vi "From CSV File.vi"(8 "error in":errorcluster, 9 "Path":path, 10 "engine in":refnum<class "engine configuration.lvclass">, 11 "SystemLink editor node in":refnum<class "SystemLink File editor node.lvclass">) -> (0 "error out":errorcluster, 1 "Update":bool, 2 "engine out":refnum<class "engine configuration.lvclass">, 3 "SystemLink editor node out":refnum<class "SystemLink File editor node.lvclass">)   [LabVIEW 2015, in "SystemLink File editor node.lvclass"]
uses:
  SystemLink File editor node.lvclass
  <vilib>/NI/Configuration Framework/serializable configuration/NISE_CEF_serializable configuration.lvclass
  <vilib>/NI/Module Execution Interface/Engine Configuration/engine configuration.lvclass
  <vilib>/NI/Tag Bus/tag/tag descriptor.lvclass
  module/configuration/SystemLink File configuration.lvclass
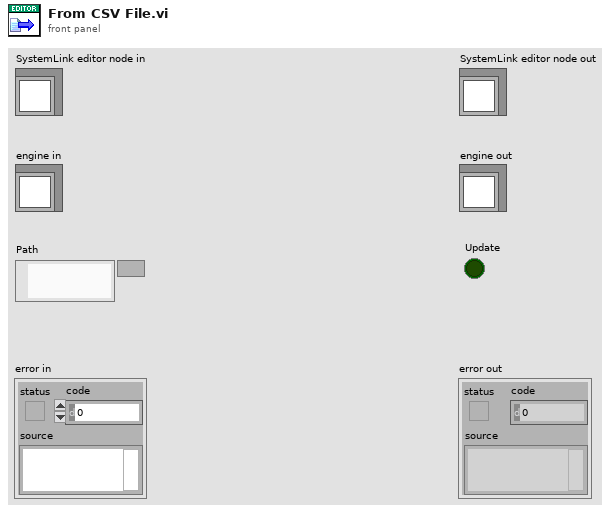
[diagram p1: front panel]
types:
  T1 = typedef "SystemLink File configuration.lvclass/Line.ctl" = cluster{"channel":refnum<class "TBM channel.lvclass">, "Data Tag Type":T2}
  T2 = typedef "SystemLink File configuration.lvclass/Data Tag Type.ctl" = enum16{"Double", "Single", "I32", "I16", "I8", "U64", "U32", "U16", "U8", "Boolean", "String", "Timestamp"}
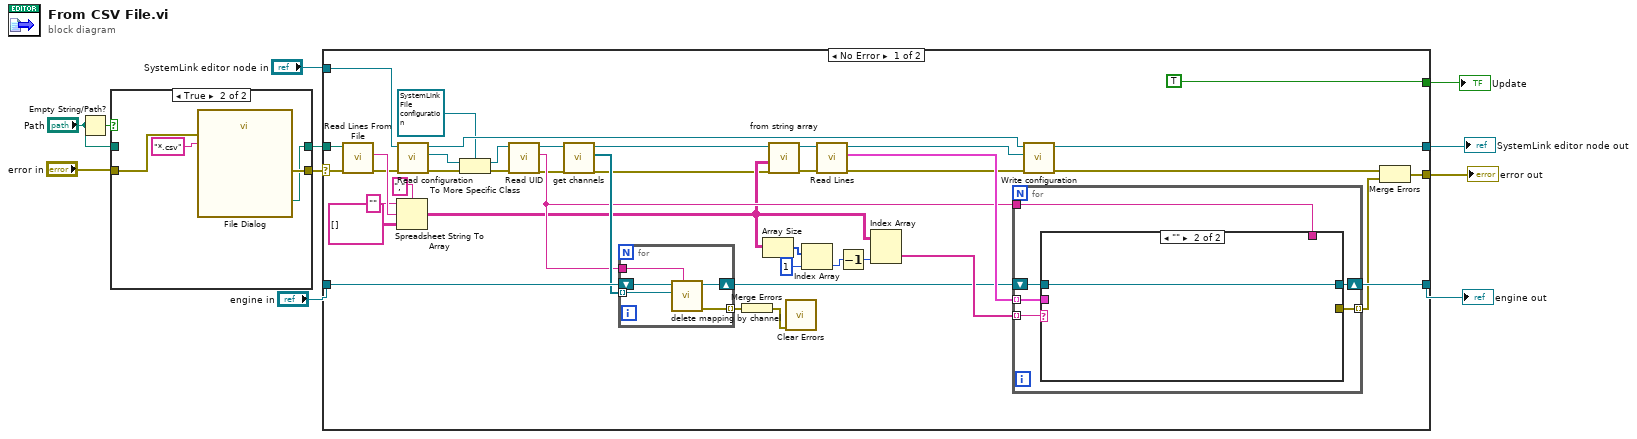
[diagram p0: block diagram]
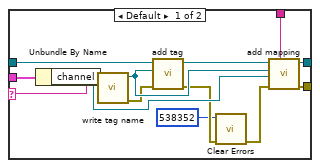
[diagram p3: hidden frame]
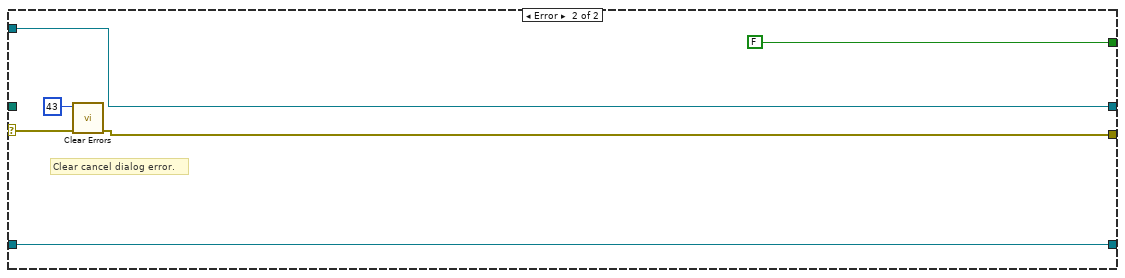
[diagram p4: hidden frame]
diagram:
  n1 = Empty String/Path?(string/path="Path") -> (empty?=w5:bool)
  n2 = case shown="True" w5 {
    tunnel: "error in" -> [w12 w16]
    tunnel: [w12 w15] -> w3
    tunnel: [w13 w14] -> w2
    tunnel: "Path" -> [w13 _]
    frame False {
    }
    frame True {
      n3 = call "File Dialog"("error in"=w16, "pattern (all files)"="*.csv") -> ("selected path"=w14:path, "error out"=w15:errorcluster)  [unwired: 10 in, 2 out]
    }
  }
  n4 = case shown="No Error" w3 {
    selector: w3 -> [w51 w86]
    tunnel: [w36 w85] -> w8
    tunnel: [w22 w88] -> w10
    tunnel: "SystemLink editor node in" -> [w29 w88]
    tunnel: w2 -> [w56 _]
    tunnel: [TRUE ("Update") FALSE ("Update")] -> w11
    tunnel: "engine in" -> [w48 w83]
    tunnel: [w39 w83] -> w9
    frame No Error {
      n5 = call <vilib>:"Read Lines From File.vi"("file path (dialog if empty)"=w56, "error in (not an error)"=w51) -> ("line string"=w54:string, "error out"=w28:errorcluster)  [unwired: 5 in, 1 out]
      n6 = Spreadsheet String To Array(delimiter (Tab)=",", format string="", spreadsheet string=w54, array type (2D Dbl)=string[][] [] ("type (empty)")) -> (array=w34:string[][])
      n7 = call-dynamic "Read configuration.vi"("error in"=w28, "SystemLin Tag Module editor node in"=w29) -> ("error out"=w26:errorcluster, "configuration"=w27:refnum<class "NISE_CEF_serializable configuration.lvclass">, "SystemLin Tag Module editor node out"=w25:refnum<class "SystemLink File editor node.lvclass">)  [unwired: 7 in]
      n8 = To More Specific Class(target class=refnum<class "SystemLink File configuration.lvclass"> refnum ("SystemLin Tag Module configuration"), reference=w27, error in=w26) -> (specific class reference=w50:refnum<class "SystemLink File configuration.lvclass">, error out=w44:errorcluster)
      n9 = call <vilib>:"Read UID.vi"("error in"=w44, "configuration in"=w50) -> ("error out"=w19:errorcluster, "instance id"=w37:string, "configuration out"=w49:refnum<class "SystemLink File configuration.lvclass">)  [unwired: 7 in]
      n10 = call-dynamic "get channels.vi"("SystemLin Tag Module configuration in"=w49) -> ("channels"=w47:refnum<class "TBM channel.lvclass">[], "SystemLin Tag Module configuration out"=w45:refnum<class "SystemLink File configuration.lvclass">)  [unwired: 9 in]
      n11 = for {
        tunnel: w37 -> [w81]
        tunnel: w47 -> [w80] mode=indexing
        tunnel: [w79] -> w46 mode=indexing
        shift-right: [w78] -> w40
        shift-left: w48 -> [w82]
        n12 = call <vilib>:"delete mapping by channel.vi"("owner ID"=w81, "channel"=w80, "engine configuration in"=w82) -> ("error out"=w79:errorcluster, "engine configuration out"=w78:refnum<class "engine configuration.lvclass">)  [unwired: 7 in]
      }
      n13 = Merge Errors(w46) -> (w20:errorcluster)
      n14 = Array Size(array=w34) -> (size(s)=w33:i32[])
      n15 = call-dynamic "from string array.vi"("error in (no error)"=w19, "String Array"=w34, "module configuration in"=w45) -> ("error out"=w38:errorcluster, "module configuration out"=w43:refnum<class "SystemLink File configuration.lvclass">)  [unwired: 7 in]
      n16 = call <vilib>:"Clear Errors.vi"("error in (no error)"=w20) -> ()  [unwired: 5 in, 2 out]
      n17 = Index Array(array=w33, index=1) -> (element=w31:i32)
      n18 = call "Read Lines.vi"("error in (no error)"=w38, "SystemLin Tag Module configuration in"=w43) -> ("error out"=w23:errorcluster, "Lines"=w42:T1[], "SystemLin Tag Module configuration out"=w24:refnum<class "SystemLink File configuration.lvclass">)  [unwired: 7 in]
      n19 = Decrement(x=w31) -> (x-1=w30:i32)
      n20 = Index Array(array=w34, index (col)=w30) -> (element=w41:string[])  [unwired: 1 in]
      n21 = for {
        tunnel: w42 -> [w63] mode=indexing
        tunnel: w41 -> [w58] mode=indexing
        shift-right: [w62] -> w39
        shift-left: w40 -> [w59]
        tunnel: w37 -> [w61]
        tunnel: [w60] -> w35 mode=indexing
        n22 = case shown="\"\"" w58 {
          selector: w58 -> [w64 _]
          tunnel: w63 -> [w76 _]
          tunnel: [w75 w77] -> w62
          tunnel: w61 -> [w74 _]
          tunnel: [w73 _] -> w60
          tunnel: w59 -> [w72 w77]
          frame Default {
            n23 = Unbundle By Name(w76) -> ("channel"=w69:refnum<class "TBM channel.lvclass">)
            n24 = call <vilib>:"write tag name.vi"("name"=w64, "system tag in"=w69) -> ("error out"=w68:errorcluster, "system tag out"=w70:refnum<class "TBM channel.lvclass">)  [unwired: 8 in]
            n25 = call-dynamic "add tag.vi"("error in"=w68, "tag descriptor"=w70, "engine configuration in"=w72) -> ("error out"=w67:errorcluster, "engine configuration out"=w71:refnum<class "engine configuration.lvclass">)  [unwired: 7 in]
            n26 = call <vilib>:"Clear Errors.vi"("error in (no error)"=w67, "specific error code to clear (0: all)"=538352) -> ("error out"=w66:errorcluster)  [unwired: 4 in, 1 out]
            n27 = call-dynamic "add mapping.vi"("owner ID"=w74, "error in"=w66, "channel"=w69, "tag descriptor"=w70, "engine configuration"=w71) -> ("error out"=w73:errorcluster, "engine configuration out"=w75:refnum<class "engine configuration.lvclass">)  [unwired: 5 in]
          }
          frame "" {
          }
        }
      }
      n28 = call-dynamic "Write configuration.vi"("error in"=w23, "configuration"=w24, "SystemLin Tag Module editor node in"=w25) -> ("error out"=w21:errorcluster, "SystemLin Tag Module editor node out"=w22:refnum<class "SystemLink File editor node.lvclass">)  [unwired: 7 in]
      n29 = Merge Errors(w21, w35) -> (w36:errorcluster)
    }
    frame Error {
      # "Clear cancel dialog error."
      n30 = call <vilib>:"Clear Errors.vi"("error in (no error)"=w86, "specific error code to clear (0: all)"=43) -> ("error out"=w85:errorcluster)  [unwired: 4 in, 1 out]
    }
  }
  "error out" <- w8
  "SystemLink editor node out" <- w10
  "Update" <- w11
  "engine out" <- w9
